vi "subTruncateFilterCplxClstr.vi"(1 "samples per symbol (16)":i32, 2 "filter length (symbols)":i32, 3 "waveform to truncate":T1 caption="input complex waveform" {"Y" format="%.3f"; "dt" format="%^.2e"; "t0" format="%.4f"}) -> (0 "truncated waveform":T1 caption="output complex waveform" {"Y" format="%.3f"; "dt" format="%^.2e"; "t0" format="%.4f"})   [LabVIEW 2019]
uses:
  <vilib>/addons/Modulation/Analog/controls/Complex Data Waveform.ctl
  <vilib>/addons/Modulation/niAMT.lvlib
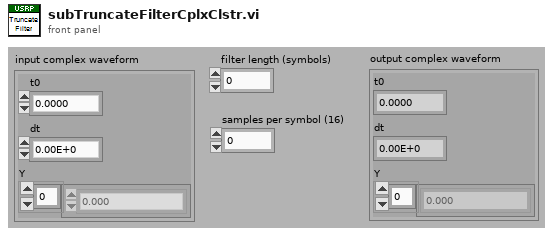
[diagram p1: front panel]
types:
  T1 = typedef "niAMT.lvlib/Complex Data Waveform.ctl" = cluster{"t0":dbl, "dt":dbl, "Y":cdb[]}
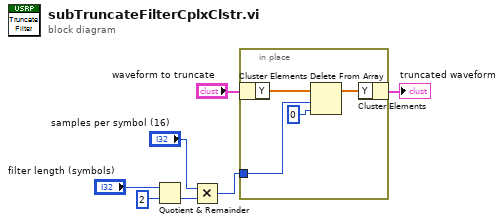
[diagram p0: block diagram]
diagram:
  n1 = Quotient & Remainder(x="filter length (symbols)", y=2) -> (floor(x/y)=w1:i32)  [unwired: 1 out]
  n2 = Multiply(x="samples per symbol (16)", y=w1) -> (x*y=w4:i32)
  n3 = in-place {
    in-place-border: w4 -> [w11]
    n4 = in-place-cluster #1("waveform to truncate") -> ("Y"=w8:cdb[])
    n5 = Delete From Array(array=w8, length=w11, index=0) -> (array with subset deleted=w9:cdb[])  [unwired: 1 out]
    n6 = in-place-cluster #1("Y"=w9) -> (→"truncated waveform":T1)
  }
